vi "Constants.vi"() -> ()   [LabVIEW 2019, in "Diagnostics Addon Shared.lvlib"]
doc: "Use this Global VI to access the GUIDs assigned to the page resources of the Custom Device."
uses:
  Diagnostics Addon Shared.lvlib
panel:
  in  "Tab Control":T1(tab)
  in  "Diagnostic Command CAN Connected GUID":string="1FB7B5C2-C5A9-4D5A-B9BF-360A427E9C45"
  in  "Service Channel Timestamp GUID":string="DF42C646-E0F5-4FDC-B61F-A239DDC21DB6"
  in  "Service Channel Success GUID":string="250721A4-6B94-4316-BB53-871C460EF5BF"
  in  "Service Channel Error Code GUID":string="702D1531-E61D-4E97-9600-C0343F3643DE"
  in  "Service Channel Trigger GUID":string="07620D9D-7630-47C2-94EA-6EC090C7ED25"
  in  "Addon Status GUID":string="D2E29887-53A4-41DF-A894-75F3232784D2"
  in  "Diag Functions Collection GUID":string="815D9C25-31D7-4FB4-8370-E700F2F3EFDC"
  in  "DTCs Collection GUID":string="A2A849E8-7BE4-4A2F-A1FF-31B2D896165C"
  in  "Settings Section GUID":string="776B8ED8-B501-4E9A-BC63-BC5D124AAE72"
  in  "Raw Signal GUID":string="14F7FD44-C9B7-4E77-B7DD-C791D8E28C31"
  in  "Service Channels GUID":string="7A409464-F136-4C61-8408-2BA591C10830"
  in  "Memory Output GUID":string="201256EA-AB1F-4DBE-873B-1A9BA778017B"
  in  "DID Output GUID":string="1DA85E41-B8B2-4229-BAF4-C924308D18D5"
  in  "PID Output GUID":string="414A03E8-4A35-4FB1-B7BA-356F958C107C"
  in  "Poll GUID":string="097733FF-7DEA-4C1E-9892-797683DC1715"
  in  "Polling GUID":string="4C6F8359-E716-4E90-A19A-6DD83BA7AB18"
  in  "User Defined Message GUID":string="C252BD32-0316-4CF0-8E56-317862ECDC4C"
  in  "User Defined Group GUID":string="00F9F4F4-030C-44AD-8756-214B06E3F58A"
  in  "User Defined GUID":string="CFA7BF4B-764C-45FB-BBED-38F184212CC0"
  in  "DID Outputs GUID":string="a1b4f299-b02f-4aee-83c4-b2663edfc3d0"
  in  "DTC Control GUID":string="c7c1a7e9-77d4-474c-a0e9-38edab0be724"
  in  "Memory Input GUID":string="bcff0b3d-7243-4886-a340-96f6fb52a52d"
  in  "Memory Inputs GUID":string="09bcd3f1-7ebd-43d6-9f90-c7b275b290a5"
  in  "Memory Outputs GUID":string="8568ba9d-faad-4aba-a1fa-a7191ea76f8f"
  in  "Memory GUID":string="ddf9fde4-b7c4-46c2-b039-1cf8b908c912"
  in  "DID Inputs GUID":string="7aa10d41-82af-42f0-a422-22627e0c3946"
  in  "Diagnostics_Enable":string="0B9E0FC8-0CF3-4008-BFB5-1E927C310F03"
  in  "Read DTCs GUID":string="631db7b8-0b52-4af9-934d-144228c2dbd8"
  in  "PIDs GUID":string="1514cba4-fa1e-47dd-8223-616adb9fb21d"
  in  "Commands GUID":string="14802196-9eef-416a-8ce6-e6467da1d504"
  in  "PID Input GUID":string="6b934904-49a9-4798-a421-a2da3be45ca1"
  in  "PID Inputs GUID":string="3a9eaf02-736d-4e36-bf88-b98c7e9eb737"
  in  "DPIDs GUID":string="186cc3e9-a602-40ff-b933-3b68f6fbfaf8"
  in  "DPID GUID":string="be84dd52-6fa5-4162-93da-bfddf126599b"
  in  "DTC GUID":string="7ba6be2c-4857-4b46-8446-f293283a3924"
  in  "Diagnostics_Disable":string="F25C602E-152F-45E8-8766-09738EB15F4F"
  in  "PID Outputs GUID":string="edf3a6ba-361e-4d29-8f85-616268b5a338"
  in  "IO GUID":string="340d50a8-4c77-4b9c-9e2b-69668480a08c"
  in  "Routine GUID":string="6fce7018-00fd-4fe4-bfd5-c0801fde7f06"
  in  "Signal GUID":string="813ed40a-6aa8-4ff9-92f7-887fb6dec76c"
  in  "Protected Signal GUID":string="edc2e041-ff43-4610-a968-1d89a067df1d"
  in  "DID Input GUID":string="465d9377-cb59-4ae9-97ed-bc842761823f"
  in  "Routine Start GUID":string="7299a859-e27a-4f6d-ab3a-db802fb4db39"
  in  "Routine Stop GUID":string="77ae2b93-bc49-4a11-9803-49f6a1a61766"
  in  "Routine Request GUID":string="ed43eaed-92e2-4ea6-9195-de19bee607ee"
  in  "IO Controls GUID":string="0ac6196a-385b-4d7f-b227-6021e7d2e1e7"
  in  "Routines GUID":string="0ff37a6c-fd65-46dd-8b75-df84d7ab3dd8"
  in  "Response GUID":string="bc55b15e-e331-4782-b5d4-23fb44f573db"
  in  "Command GUID":string="37a28eab-899c-4060-83a1-bccb94c61935"
  in  "DIDs GUID":string="ae6faf55-1aff-4d2a-b6e8-d238aa342751"
  in  "Command Channel GUID":string="8838CE65-E521-4441-9757-12B25FC7A11C"
  in  "Diag CAN Control GUID":string="9B8C8DBD-2385-4800-B95A-DC5808FA6AFE"
  in  "Service Response GUID":string="2FD9705E-A3C4-4FDD-BCC4-9A14EB459DC7"
  in  "Service Command GUID":string="CD4ADA30-2AAD-4769-A327-34E422452A7D"
  in  "Tester Present GUID":string="C61DB15D-6FF4-4348-8893-8D4ED8FDE67C"
  in  "Clear DTCs GUID":string="48C6923E-40FF-4AB6-92F2-B52C58569929"
  in  "DTC Change Count GUID":string="63AF7131-6C63-46E9-8B55-FCC1ADF5433D"
  in  "Unlock ECU GUID":string="CC186E36-917D-4B89-B851-45BBEB39AAD6"
  in  "Reset ECU GUID":string="802F25CA-C7EB-41D9-AB2D-B1D032A724A3"
  in  "Diagnostic Session Control GUID":string="CEADB72E-B742-4D35-B124-F9CB7CB35587"
  in  "Normal Communication Control GUID":string="49358E36-D7EF-421D-B92B-812ACD41B7AE"
  in  "Master Key Byte Length":string="Master Key Byte Length"
  in  "Master Key":string="Master Key"
  in  "Addon Status":string="Addon Status"
  in  "Service Channel Success":string="Success"
  in  "Error Codes":cluster{"Code":i32, "String":string}[](array[cluster])=[{"Code"=0, "String"="<0> No Error."}, {"Code"=8000, "String"="<8000> The selected arbitration ID is already in the list of filtered arbitration IDs."}, {"Code"=8001, "String"="<8001> A read buffer in the driver or the software overflowed and surplus data may have been dropped. Other high-priority tasks might be using excessive system resources."}, {"Code"=-8000, "String"="<-8000> The handle passed to the function is not valid."}, {"Code"=1, "String"="<1> The selected CAN interface is already active using different settings."}, {"Code"=2, "String"="<2> Diagnostic protocol timeout. A response from the ECU was not received."}, {"Code"=3, "String"="<3> The arbitration ID passed to the function is not valid."}, {"Code"=4, "String"="<4> An internal timeout occurred."}, {"Code"=5, "String"="<5> A required hardware driver support library could not be loaded. Verify that the requested driver is installed or refer to product documentation about specifying the correct driver."}, {"Code"=6, "String"="<6> The name of the interface is not valid."}, {"Code"=7, "String"="<7> The function called is not supported."}, {"Code"=8, "String"="<8> A parameter passed to the function is not valid."}, {"Code"=9, "String"="<9> The selected property is not defined."}, {"Code"=10, "String"="<10> The selected property is read only."}, {"Code"=11, "String"="<11> A callback function has already been defined. To define another callback function, clear the active callback first."}, {"Code"=12, "String"="<12> The function called is not implemented in the nibci.dll. Please update the nibci.dll to a newer version."}, {"Code"=13, "String"="<13> The supplied FPGA bit file is missing one or more mandatory interface elements. Please make sure that your FPGA logic implements the required bridge functionality."}, {"Code"=14, "String"="<14> The selected FPGA bit file was not found. Ensure it is present in the specified directory on the RT target and that you are using the correct path delimiter for the target's operating system."}, {"Code"=17, "String"="<17> The diagnostic service is unknown to the ECU."}, {"Code"=18, "String"="<18> The subfunction of the diagnostic service is unknown to the ECU (invalid format)."}, {"Code"=19, "String"="<19> The length of the request message or the format of the parameters does not match the prescribed requirements for the requested service."}, {"Code"=20, "String"="<20> The response message is too long to be transported via the network."}, {"Code"=33, "String"="<33> The diagnostic service could temporarily not be executed due to other activities (repeat request)."}, {"Code"=34, "String"="<34> The diagnostic service could not be executed due to incorrect conditions (request sequence error)."}, {"Code"=35, "String"="<35> The diagnostic service could not be executed because another function is active (routine not complete)."}, {"Code"=36, "String"="<36> The requested service is out-of-sequence. The ECU expects a different order of the requests issued."}, {"Code"=37, "String"="<37> A gateway reports that a subnet component did not respond."}, {"Code"=38, "String"="<38> A DTC is preventing the service from being executed in the ECU."}, {"Code"=49, "String"="<49> Parameter range error in diagnostic service request."}, {"Code"=51, "String"="<51> The diagnostic service could not be executed due to insufficient security privileges (security access denied)."}, {"Code"=53, "String"="<53> An invalid security key was specified to the ECU."}, {"Code"=54, "String"="<54> The diagnostic service was attempted too often (exceeds number of attempts)."}, {"Code"=55, "String"="<55> The diagnostic service was attempted too quickly (required time delay not expired)."}, {"Code"=112, "String"="<112> Upload/download to the ECU is prevented by a fault condition in the ECU."}, {"Code"=113, "String"="<113> The data transfer operation was aborted due to a fault condition in the ECU."}, {"Code"=114, "String"="<114> The ECU detected an error while erasing or programming its memory (general programming failure)."}, {"Code"=115, "String"="<115> The ECU detected an error in the sequence of block sequence counter values during data transfer."}, {"Code"=126, "String"="<126> The subfunction of the diagnostic service is not supported in the active diagnostic session."}, {"Code"=127, "String"="<127> The diagnostic service is not supported in the active diagnostic session."}, {"Code"=128, "String"="<128> The ECU returned manufacturer specific error code 128."}, {"Code"=129, "String"="<129> The ECU returned manufacturer specific error code 129."}, {"Code"=130, "String"="<130> The ECU returned manufacturer specific error code 130."}, {"Code"=131, "String"="<131> The ECU returned manufacturer specific error code 131."}, {"Code"=132, "String"="<132> The ECU returned manufacturer specific error code 132."}, {"Code"=133, "String"="<133> The ECU returned manufacturer specific error code 133."}, {"Code"=134, "String"="<134> The ECU returned manufacturer specific error code 134."}, {"Code"=135, "String"="<135> The ECU returned manufacturer specific error code 135."}, {"Code"=136, "String"="<136> The ECU returned manufacturer specific error code 136."}, {"Code"=137, "String"="<137> The ECU returned manufacturer specific error code 137."}, {"Code"=138, "String"="<138> The ECU returned manufacturer specific error code 138."}, {"Code"=139, "String"="<139> The ECU returned manufacturer specific error code 139."}, {"Code"=140, "String"="<140> The ECU returned manufacturer specific error code 140."}, {"Code"=141, "String"="<141> The ECU returned manufacturer specific error code 141."}, {"Code"=142, "String"="<142> The ECU returned manufacturer specific error code 142."}, {"Code"=143, "String"="<143> The ECU returned manufacturer specific error code 143."}, {"Code"=144, "String"="<144> The ECU returned manufacturer specific error code 144."}, {"Code"=145, "String"="<145> The ECU returned manufacturer specific error code 145."}, {"Code"=146, "String"="<146> The ECU returned manufacturer specific error code 146."}, {"Code"=147, "String"="<147> The ECU returned manufacturer specific error code 147."}, {"Code"=148, "String"="<148> The ECU returned manufacturer specific error code 148."}, {"Code"=149, "String"="<149> The ECU returned manufacturer specific error code 149."}, {"Code"=150, "String"="<150> The ECU returned manufacturer specific error code 150."}, {"Code"=-8256, "String"="<-8256> Invalid frame received by transport layer."}, {"Code"=-8257, "String"="<-8257> Out-of-sequence frame received by transport layer."}, {"Code"=-8258, "String"="<-8258> Transmit aborted by transport layer due to overflow in the receiver."}, {"Code"=-8259, "String"="<-8259> Transmit aborted by transport layer (maximum wait frames received)."}, {"Code"=-8260, "String"="<-8260> Diagnostic command timeout. A response from the ECU was not received."}, {"Code"=-8261, "String"="<-8261> ISO TP: timeout receiving a Consecutive Frame."}, {"Code"=-8262, "String"="<-8262> ISO TP: timeout receiving a Flow Control Frame."}, {"Code"=-8263, "String"="<-8263> Transport protocol read timeout. A response from the ECU was not received."}, {"Code"=-8264, "String"="<-8264> VW TP 2.0 Protocol error. The selected application type is not supported by the ECU."}, {"Code"=-8265, "String"="<-8265> VW TP 2.0 Protocol error. The selected application type is temporarily not supported by the ECU."}, {"Code"=-8266, "String"="<-8266> VW TP 2.0 Protocol error. There are temporarily no resources available on the ECU."}, {"Code"=-8267, "String"="<-8267> VW TP 2.0 Protocol error. An invalid response was received from the ECU."}, {"Code"=-8268, "String"="<-8268> VW TP 2.0 not initialized. Call 'VWTP TP-Request.vi' before calling this VI."}, {"Code"=-8269, "String"="<-8269> Receive aborted with OVERLOAD frame due to user settings."}, {"Code"=-8270, "String"="<-8270> Invalid response message received."}, {"Code"=-8300, "String"="<-8300> DoIP (Diagnostic on Internet Protocol): Transmitted message truncated."}, {"Code"=-8301, "String"="<-8301> DoIP (Diagnostic on Internet Protocol): Incorrect target address received."}, {"Code"=-8302, "String"="<-8302> DoIP (Diagnostic on Internet Protocol): Incorrect source address received."}, {"Code"=-8306, "String"="<-8306> DoIP (Diagnostic on Internet Protocol): Generic header error received."}, {"Code"=-8344, "String"="<-8344> DoIP (Diagnostic on Internet Protocol): Routing activation response: Routing activation denied due to unsupported routing activation type."}, {"Code"=-8345, "String"="<-8345> DoIP (Diagnostic on Internet Protocol): Routing activation response: Routing activation denied due to confirmation rejected."}, {"Code"=-8346, "String"="<-8346> DoIP (Diagnostic on Internet Protocol): Routing activation response: Routing activation denied due to missing authentication."}, {"Code"=-8347, "String"="<-8347> DoIP (Diagnostic on Internet Protocol): Routing activation response: Routing activation denied because the SA is already registered and active on a different TCP_DATA socket."}, {"Code"=-8348, "String"="<-8348> DoIP (Diagnostic on Internet Protocol): Routing activation response: Routing activation denied because an SA different from the table connection entry was received on the already activated TCP_DATA socket."}, {"Code"=-8349, "String"="<-8349> DoIP (Diagnostic on Internet Protocol): Routing activation response: Routing activation denied because all concurrently supported TCP_DATA sockets are registered and active."}, {"Code"=-8350, "String"="<-8350> DoIP (Diagnostic on Internet Protocol): Routing activation response: Routing activation denied due to unknown source address."}, {"Code"=-8352, "String"="<-8352> DoIP (Diagnostic on Internet Protocol): Routing activation response: OEM specific message 254."}, {"Code"=-8353, "String"="<-8353> DoIP (Diagnostic on Internet Protocol): Routing activation response: OEM specific message 253."}, {"Code"=-8354, "String"="<-8354> DoIP (Diagnostic on Internet Protocol): Routing activation response: OEM specific message 252."}, {"Code"=-8355, "String"="<-8355> DoIP (Diagnostic on Internet Protocol): Routing activation response: OEM specific message 251."}, {"Code"=-8356, "String"="<-8356> DoIP (Diagnostic on Internet Protocol): Routing activation response: OEM specific message 250."}, {"Code"=-8357, "String"="<-8357> DoIP (Diagnostic on Internet Protocol): Routing activation response: OEM specific message 249."}, {"Code"=-8358, "String"="<-8358> DoIP (Diagnostic on Internet Protocol): Routing activation response: OEM specific message 248."}, {"Code"=-8359, "String"="<-8359> DoIP (Diagnostic on Internet Protocol): Routing activation response: OEM specific message 247."}, {"Code"=-8360, "String"="<-8360> DoIP (Diagnostic on Internet Protocol): Routing activation response: OEM specific message 246."}, {"Code"=-8361, "String"="<-8361> DoIP (Diagnostic on Internet Protocol): Routing activation response: OEM specific message 245."}, {"Code"=-8362, "String"="<-8362> DoIP (Diagnostic on Internet Protocol): Routing activation response: OEM specific message 244."}, {"Code"=-8363, "String"="<-8363> DoIP (Diagnostic on Internet Protocol): Routing activation response: OEM specific message 243."}, {"Code"=-8364, "String"="<-8364> DoIP (Diagnostic on Internet Protocol): Routing activation response: OEM specific message 242."}, {"Code"=-8365, "String"="<-8365> DoIP (Diagnostic on Internet Protocol): Routing activation response: OEM specific message 241."}, {"Code"=-8366, "String"="<-8366> DoIP (Diagnostic on Internet Protocol): Routing activation response: OEM specific message 240."}, {"Code"=-8367, "String"="<-8367> DoIP (Diagnostic on Internet Protocol): Routing activation response: OEM specific message 239."}, {"Code"=-8368, "String"="<-8368> DoIP (Diagnostic on Internet Protocol): Routing activation response: OEM specific message 238."}, {"Code"=-8369, "String"="<-8369> DoIP (Diagnostic on Internet Protocol): Routing activation response: OEM specific message 237."}, {"Code"=-8370, "String"="<-8370> DoIP (Diagnostic on Internet Protocol): Routing activation response: OEM specific message 236."}, {"Code"=-8371, "String"="<-8371> DoIP (Diagnostic on Internet Protocol): Routing activation response: OEM specific message 235."}, {"Code"=-8372, "String"="<-8372> DoIP (Diagnostic on Internet Protocol): Routing activation response: OEM specific message 234."}, {"Code"=-8373, "String"="<-8373> DoIP (Diagnostic on Internet Protocol): Routing activation response: OEM specific message 233."}, {"Code"=-8374, "String"="<-8374> DoIP (Diagnostic on Internet Protocol): Routing activation response: OEM specific message 232."}, {"Code"=-8375, "String"="<-8375> DoIP (Diagnostic on Internet Protocol): Routing activation response: OEM specific message 231."}, {"Code"=-8376, "String"="<-8376> DoIP (Diagnostic on Internet Protocol): Routing activation response: OEM specific message 230."}, {"Code"=-8377, "String"="<-8377> DoIP (Diagnostic on Internet Protocol): Routing activation response: OEM specific message 229."}, {"Code"=-8378, "String"="<-8378> DoIP (Diagnostic on Internet Protocol): Routing activation response: OEM specific message 228."}, {"Code"=-8379, "String"="<-8379> DoIP (Diagnostic on Internet Protocol): Routing activation response: OEM specific message 227."}, {"Code"=-8380, "String"="<-8380> DoIP (Diagnostic on Internet Protocol): Routing activation response: OEM specific message 226."}, {"Code"=-8381, "String"="<-8381> DoIP (Diagnostic on Internet Protocol): Routing activation response: OEM specific message 225."}, {"Code"=-8382, "String"="<-8382> DoIP (Diagnostic on Internet Protocol): Routing activation response: OEM specific message 224."}, {"Code"=-8400, "String"="<-8400> DoIP (Diagnostic on Internet Protocol): Incorrect diagnostic message response received."}, {"Code"=-8402, "String"="<-8402> DoIP (Diagnostic on Internet Protocol): Diagnostic message negative ACK: Invalid source address."}, {"Code"=-8403, "String"="<-8403> DoIP (Diagnostic on Internet Protocol): Diagnostic message negative ACK: Unknown target address."}, {"Code"=-8404, "String"="<-8404> DoIP (Diagnostic on Internet Protocol): Diagnostic message negative ACK: Diagnostic message too large."}, {"Code"=-8405, "String"="<-8405> DoIP (Diagnostic on Internet Protocol): Diagnostic message negative ACK: Out of memory."}, {"Code"=-8406, "String"="<-8406> DoIP (Diagnostic on Internet Protocol): Diagnostic message negative ACK: Target unreachable."}, {"Code"=-8407, "String"="<-8407> DoIP (Diagnostic on Internet Protocol): Diagnostic message negative ACK: Unknown network."}, {"Code"=-8408, "String"="<-8408> DoIP (Diagnostic on Internet Protocol): Diagnostic message negative ACK: Transport protocol error."}, {"Code"=-8409, "String"="<-8409> An internal error occurred."}, {"Code"=-8465, "String"="<-8465> A third-party CAN driver reported an error. Verify your settings and hardware configuration"}, {"Code"=-8466, "String"="<-8466> An unexpected error occurred in the BCI layer."}, {"Code"=-8467, "String"="<-8467> The interface device reported a critical error. Data may have been lost or corrupted."}, {"Code"=8468, "String"="<8468> A read buffer in the driver or the software overflowed and surplus data may have been dropped. Other high-priority tasks might be using excessive system resources."}, {"Code"=-8469, "String"="<-8469> A write buffer in the driver or the software overflowed and the provided data was not transmitted. Please wait for parts of the buffer to be processed and try again."}, {"Code"=-8470, "String"="<-8470> A frame in a format invalid for the current communication mode was received or requested to be transmitted, e.g. the data size was outside of the allowed range."}, {"Code"=-8471, "String"="<-8471> ISO CAN FD mode is not supported for the selected interface and its installed driver version. Refer to product documentation for information about hardware and driver version support."}, {"Code"=-8472, "String"="<-8472> The driver could not be loaded for the selected NI-CAN device. Verify that the driver is installed or refer to product documentation about specifying the correct driver."}, {"Code"=-8473, "String"="<-8473> This error is currently not defined but reserved for future extensions."}, {"Code"=-8474, "String"="<-8474> This error is currently not defined but reserved for future extensions."}, {"Code"=-8475, "String"="<-8475> This error is currently not defined but reserved for future extensions."}, {"Code"=-8476, "String"="<-8476> This error is currently not defined but reserved for future extensions."}, {"Code"=-8477, "String"="<-8477> This error is currently not defined but reserved for future extensions."}, {"Code"=-8478, "String"="<-8478> This error is currently not defined but reserved for future extensions."}, {"Code"=-8479, "String"="<-8479> This error is currently not defined but reserved for future extensions."}, {"Code"=-8480, "String"="<-8480> This error is currently not defined but reserved for future extensions."}]
  in  "Enable Channel Name":string="Enable"
  in  "Poll Name":string="Poll"
  in  "DTCs Collection Page":string="DTCs"
  in  "Diag Functions Collection Page":string="Diag Functions"
  in  "Settings Page":string="Settings"
  in  "Ref.ServiceSettings":string="ServiceSettings"
  in  "Ref.ServiceChannelsStatus":string="ServiceChannelsStatus"
  in  "Service Channels Name":string="Service Channels"
  in  "Service Channel Trigger":string="Trigger"
  in  "Service Channel Error Code":string="Error Code"
  in  "Service Channel Timestamp":string="Timestamp"
  in  "Polling Name":string="Polling"
  in  "DTC_Signal Status Index":i32=2
  in  "DTC_Signal Value Index":i32=1
  in  "Diagnostic Command CAN Connected":string="CAN Connected"
  in  "Ref.CANConnected":string="CANConnected"
  in  "Ref.Triggers":string="Triggers"
  in  "Ref.Cmds":string="Cmds"
  in  "Ref.Writes":string="WriteData"
  in  "Ref.Status":string="Statuses"
  in  "Ref.DTC.Count":string="DTCCount"
  in  "Ref.DTCs":string="DTCData"
  in  "Ref.Reads":string="ReadData"
  in  "User Defined Message Name":string="Message"
  in  "User Defined Group Name":string="Group"
  in  "User Defined Name":string="User Defined"
  in  "Memory Page":string="Memory"
  in  "Response Page":string="Response"
  in  "Command Page":string="Command"
  in  "Routines Page":string="Routines"
  in  "Routine Start Page":string="Start"
  in  "Routine Stop Page":string="Stop"
  in  "Routine Request Page":string="Request"
  in  "Command Channel Name":string="Command"
  in  "DTC_Signal Suffix":string[](array[string])=["_Timestamp", "_Value", "_Status", "_Failure"]
  in  "DIDs Page":string="DIDs"
  in  "DB Alias":string="Diagnostics_Addon_Temp_DB"
  in  "DTC_Signal Prefix":string="DTC_"
  in  "Inputs Page":string="Inputs"
  in  "DPIDs Page":string="DPIDs"
  in  "LookupTableSignalsPrefix":string="SignalDefs"
  in  "LookupTableConvertPrefix":string="Convert"
  in  "PIDs Page":string="PIDs"
  in  "Read DTCs Page":string="Read DTCs"
  in  "Status Page":string="Status"
  in  "Services Page":string="Services"
  in  "Commands Page":string="Commands"
  in  "DTCs_Masks":string="DTC Masks"
  in  "Data by Identifier Page":string="Data by Identifiers"
  in  "XNETEngineSuffix":string="_XNETEngine"
  in  "ResponseQKey":string="Response"
  in  "DTCs_# of DTCs":string="Number of DTCs"
  in  "Outputs Page":string="Outputs"
  in  "IO Controls Page":string="IO Controls"
  in  "CAN.CommTimeout":string="CommTimeout"
  in  "Poll.LinkedFrames":string="Poll.LinkedFrames"
  in  "CAN.SecurityType":string="SecurityType"
  in  "DTC.Value.J2012String":string="DTC.Value.J2012String"
  in  "DTC.Status.Code":string="DTC.Status.Code"
  in  "DTC.Value.Code":string="DTC.Value.Code"
  in  "DTC.Status.String":string="DTC.Status.String"
  in  "DTC.Value.String":string="DTC.Value.String"
  in  "CAN.FDBaudRate":string="FDBaudRate"
  in  "CAN.MaxDLC":string="MaxDLC"
  in  "CAN.IOMode":string="IOMode"
  in  "LIN.NAD":string="NAD"
  in  "LIN.Cluster":string="LIN Cluster"
  in  "Type":string="Type"
  in  "CAN.Termination":string="Termination"
  in  "CAN.FillByte":string="FillByte"
  in  "CAN.FillFrame":string="FillFrame"
  in  "DTC.Order":string="ByteOrder"
  in  "DTC.AddByte":string="AddByte"
  in  "DTC.StatusByte":string="StatusByte"
  in  "DPID.PIDs":string="PIDs"
  in  "DPID.Speed":string="Speed"
  in  "Compiled.Settings":string="Compiled.Settings"
  in  "CAN.SecurityLevel":string="SecurityLevel"
  in  "CAN.SecurityDLL":string="SecurityDLL"
  in  "CAN.VWTPID":string="VWTPID"
  in  "CAN.Stream":string="Stream"
  in  "CAN.ReceiveUUDTID":string="ReceiveUUDTID"
  in  "CAN.ReceiveExt":string="ReceiveExt"
  in  "CAN.TransmitExt":string="TransmitExt"
  in  "CAN.ReceiveID":string="ReceiveID"
  in  "CAN.TransmitID":string="TransmitID"
  in  "CAN.Tranport":string="Tranport"
  in  "CAN.Protocol":string="Protocol"
  in  "CAN.BaudRate":string="BaudRate"
  in  "CAN.Interface":string="Interface"
  in  "Signal.Units":string="Units"
  in  "Signal.Name":string="Name"
  in  "Signal.DefaultValue":string="DefaultValue"
  in  "Signal.ByteOrder":string="ByteOrder"
  in  "Signal.DataType":string="DataType"
  in  "Signal.Max":string="Max"
  in  "Signal.Min":string="Min"
  in  "Signal.ScalingOffset":string="ScalingOffest"
  in  "Signal.ScalingFactor":string="ScalingFactor"
  in  "Signal.Length":string="Length"
  in  "Enable 986x":string="Enable 986x"
  in  "RIO Device 986x":string="RIO Device 986x"
  in  "RT Bitfile Location":path=path "c:/ni-rt/NIVeriStand/XNET"
  in  "Bitfile 986x":string="Bitfile 986x"
  in  "DTC.DTCByte":string="DTCByte"
  in  "ID":string="ID"
  in  "Signal.StartBit":string="StartBit"
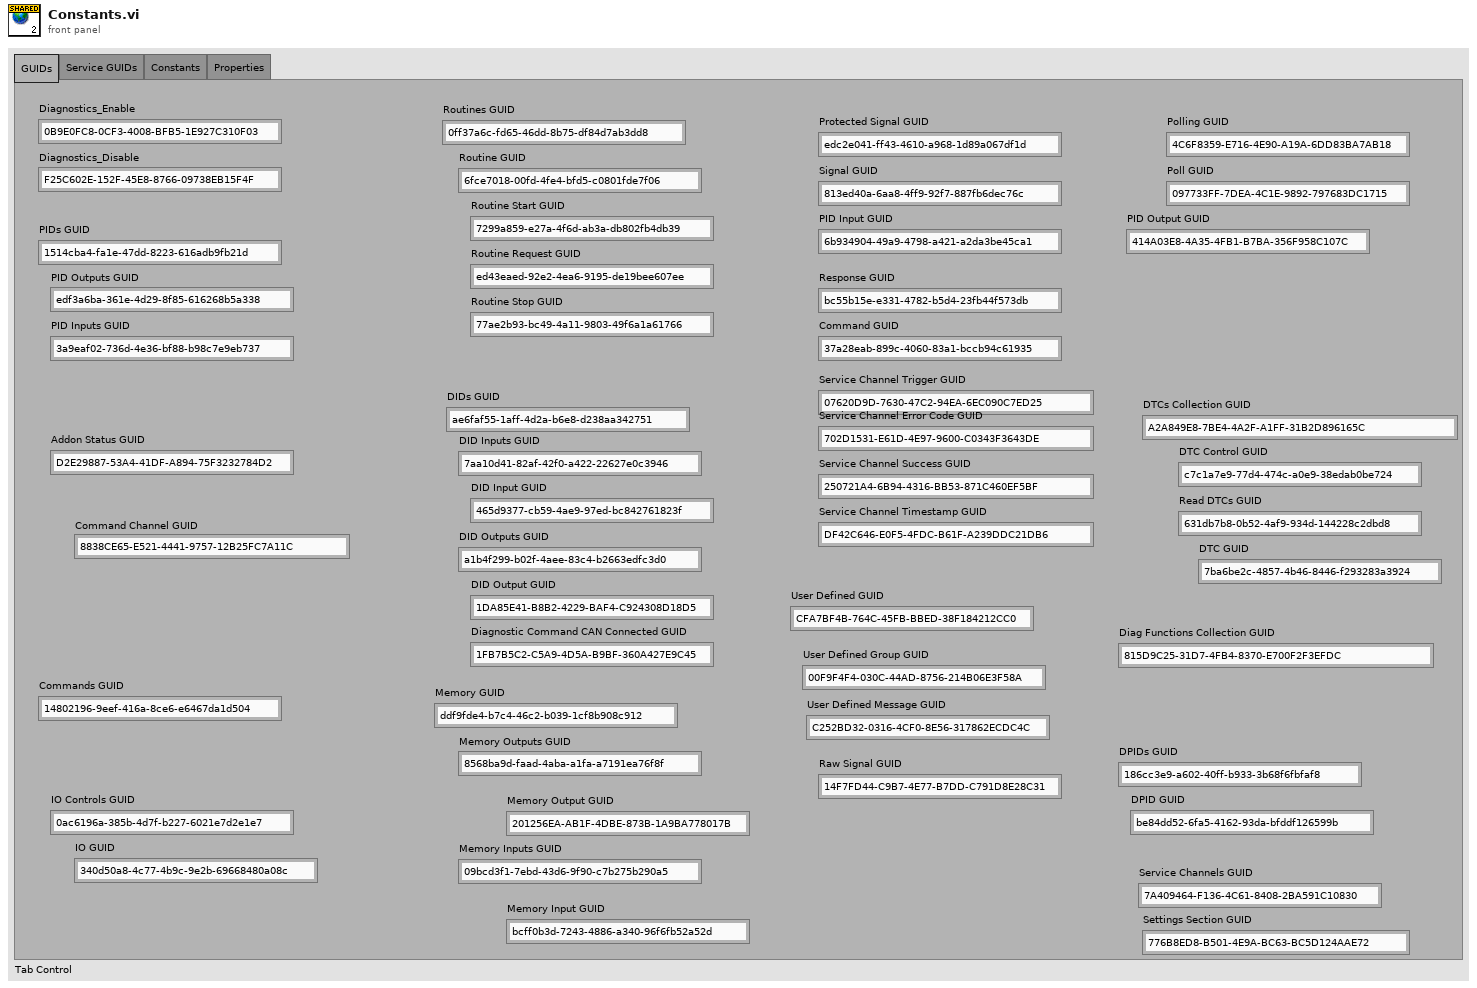
[diagram p1: front panel]
types:
  T1 = enum32{"GUIDs", "Service GUIDs", "Constants", "Properties"}
diagram:
